vi "HHMI - Count U32.vi"(7 "Reset?":bool, 10 "Increment?":bool) -> (2 "total # counted\n(Reset occurs \nprior to Increment)":u32)   [LabVIEW 2013]
doc: "Counts up. Reset returns count to zero. Increment occurs after Reset."
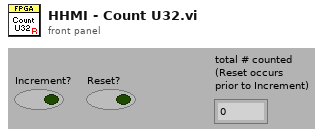
[diagram p1: front panel]
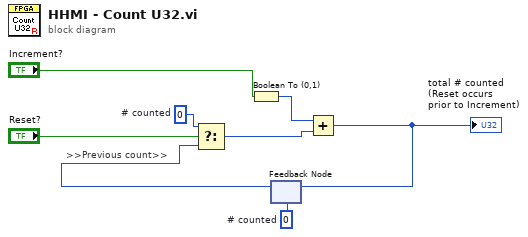
[diagram p0: block diagram]
diagram:
  w5 = u32 0  # # counted
  w8 = u32 0  # # counted
  # ">>Previous count>>"
  n1 = Boolean To (0,1)(Boolean="Increment?") -> (0, 1=w2:i16)
  n2 = feedback #1(w8) -> (w6:u32)
  n3 = Select(t=w5, s="Reset?", f=w6) -> (s? t:f=w3:u32)
  n4 = Add(x=w2, y=w3) -> (x+y=w1:u32)
  "total # counted\n(Reset occurs \nprior to Increment)" <- w1
  n5 = feedback-in #1(w1) -> ()
